vi "SimpleTCPClient.vi"(8 "error in":errorcluster, 9 "data in":string, 10 "port":u16=5001, 11 "address":string="127.0.0.1") -> (0 "error out":errorcluster)   [LabVIEW 2014]
doc: "This example VI is to be used in conjunction with the SimpleTCPServer.vi example. \nMake sure to run the SimpleTCPServer.vi prior to running this example VI otherwise an error will be generated. \n\nBoth the SimpleTCPServer.vi and SimpleTCPClient.vi can run deployed on the Raspberry Pi; the SimpleTCPServer.vi can run deployed on the Raspberry Pi and the SimpleTCPClient.vi remotely on a different networked computer or Raspberry Pi; or the SimpleTCPServer.vi can run remoterly on a different networked computer or Raspberry Pi and the SimpleTCPClient.vi deployed in the Raspberry Pi target.\n\nIf both SimpleTCPServer and SimpleTCPClient run deployed at the same Raspberry Pi, the address control value is to be left unchanged of its default 127.0.0.1 value. If the SimpleTCPClient runs on a different computer than the SimpleTCPServer example, enter the IP address of the computer running the SimpleTCPServer example in the SimpleTCPClient address control.\n\nMake sure the value of the port matches with the port value of the SimpleTCPServer vi.\n\nEnter a string message in the data in control and run the SimpleTPClient VI. Note on the running SimpleTCPServer that the remote address indicator will show the IP address of the computer where SimpleTCPClient ran. The data out indicator of SimpleTCPServer will show the same string value entered in the SimpleTCPClient data in control.\n\nTo stop the SimpleTCPServer execution, enter stop in the data in control and run SimpleTCPClient."
panel:
  in  "Stop":bool
  in  "Send Cmd":bool
  out "bytes written":i32
  # "Send stop to end"
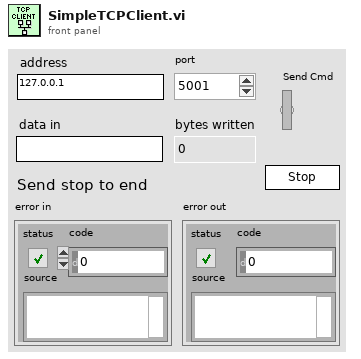
[diagram p1: front panel]
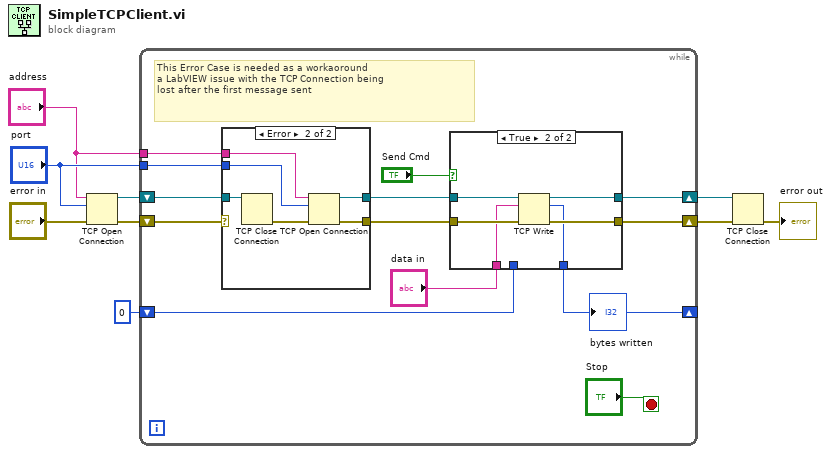
[diagram p0: block diagram]
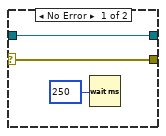
[diagram p2: hidden frame]
diagram:
  n1 = TCP Open Connection(address="address", remote port or service name="port", error in (no error)="error in") -> (connection ID=w9:refnum<k5>, error out=w8:errorcluster)  [unwired: 2 in]
  n2 = while {
    shift-right: [w22] -> w7
    shift-left: w9 -> [w16]
    shift-right: [w18] -> _
    shift-left: 0 ("bytes written") -> [w17]
    tunnel: "port" -> [w12]
    tunnel: "address" -> [w11]
    shift-right: [w21] -> w6
    shift-left: w8 -> [w15]
    stop <- "Stop" stop-if-true
    # "This Error Case is needed as a workaoround\na LabVIEW issue with the TCP Connection being\nlost after the first message sent"
    n3 = case shown="Error" w15 {
      selector: w15 -> [w24 _]
      tunnel: w16 -> [w25 w31]
      tunnel: [w25 w29] -> w14
      tunnel: [w24 w28] -> w13
      tunnel: w12 -> [_ w27]
      tunnel: w11 -> [_ w26]
      frame No Error {
        n4 = Wait (ms)(milliseconds to wait=u32 250) -> ()  [unwired: 1 out]
      }
      frame Error {
        n5 = TCP Close Connection(connection ID=w31) -> (error out=w30:errorcluster)  [unwired: 2 in, 1 out]
        n6 = TCP Open Connection(address=w26, remote port or service name=w27, error in (no error)=w30) -> (connection ID=w29:refnum<k5>, error out=w28:errorcluster)  [unwired: 2 in]
      }
    }
    n7 = case shown="True" "Send Cmd" {
      tunnel: w14 -> [w34 w40]
      tunnel: w13 -> [w33 w39]
      tunnel: "data in" -> [_ w38]
      tunnel: [w34 w37] -> w22
      tunnel: [w33 w36] -> w21
      tunnel: [w32 w35] -> w18
      tunnel: w17 -> [w32 _]
      frame False {
      }
      frame True {
        n8 = TCP Write(connection ID=w40, data in=w38, error in (no error)=w39) -> (connection ID out=w37:refnum<k5>, bytes written=w35:i32, error out=w36:errorcluster)  [unwired: 1 in]
      }
    }
    "bytes written" <- w18
  }
  n9 = TCP Close Connection(connection ID=w7, error in (no error)=w6) -> (error out=→"error out":errorcluster)  [unwired: 1 in, 1 out]
